vi "simon.vi"() -> ()   [LabVIEW 2021]
panel:
  out "Chaîne 4":string
  out "Gagné":bool
  out "Chaîne 3":string
  out "Chaîne 2":string
  in  "Cluster 3":T1
  in  "Pseudo":string
  out "Chaîne":string
  in  "Tableau":T2(array[cluster])
  in  "Tableau 3":T3(array[cluster])
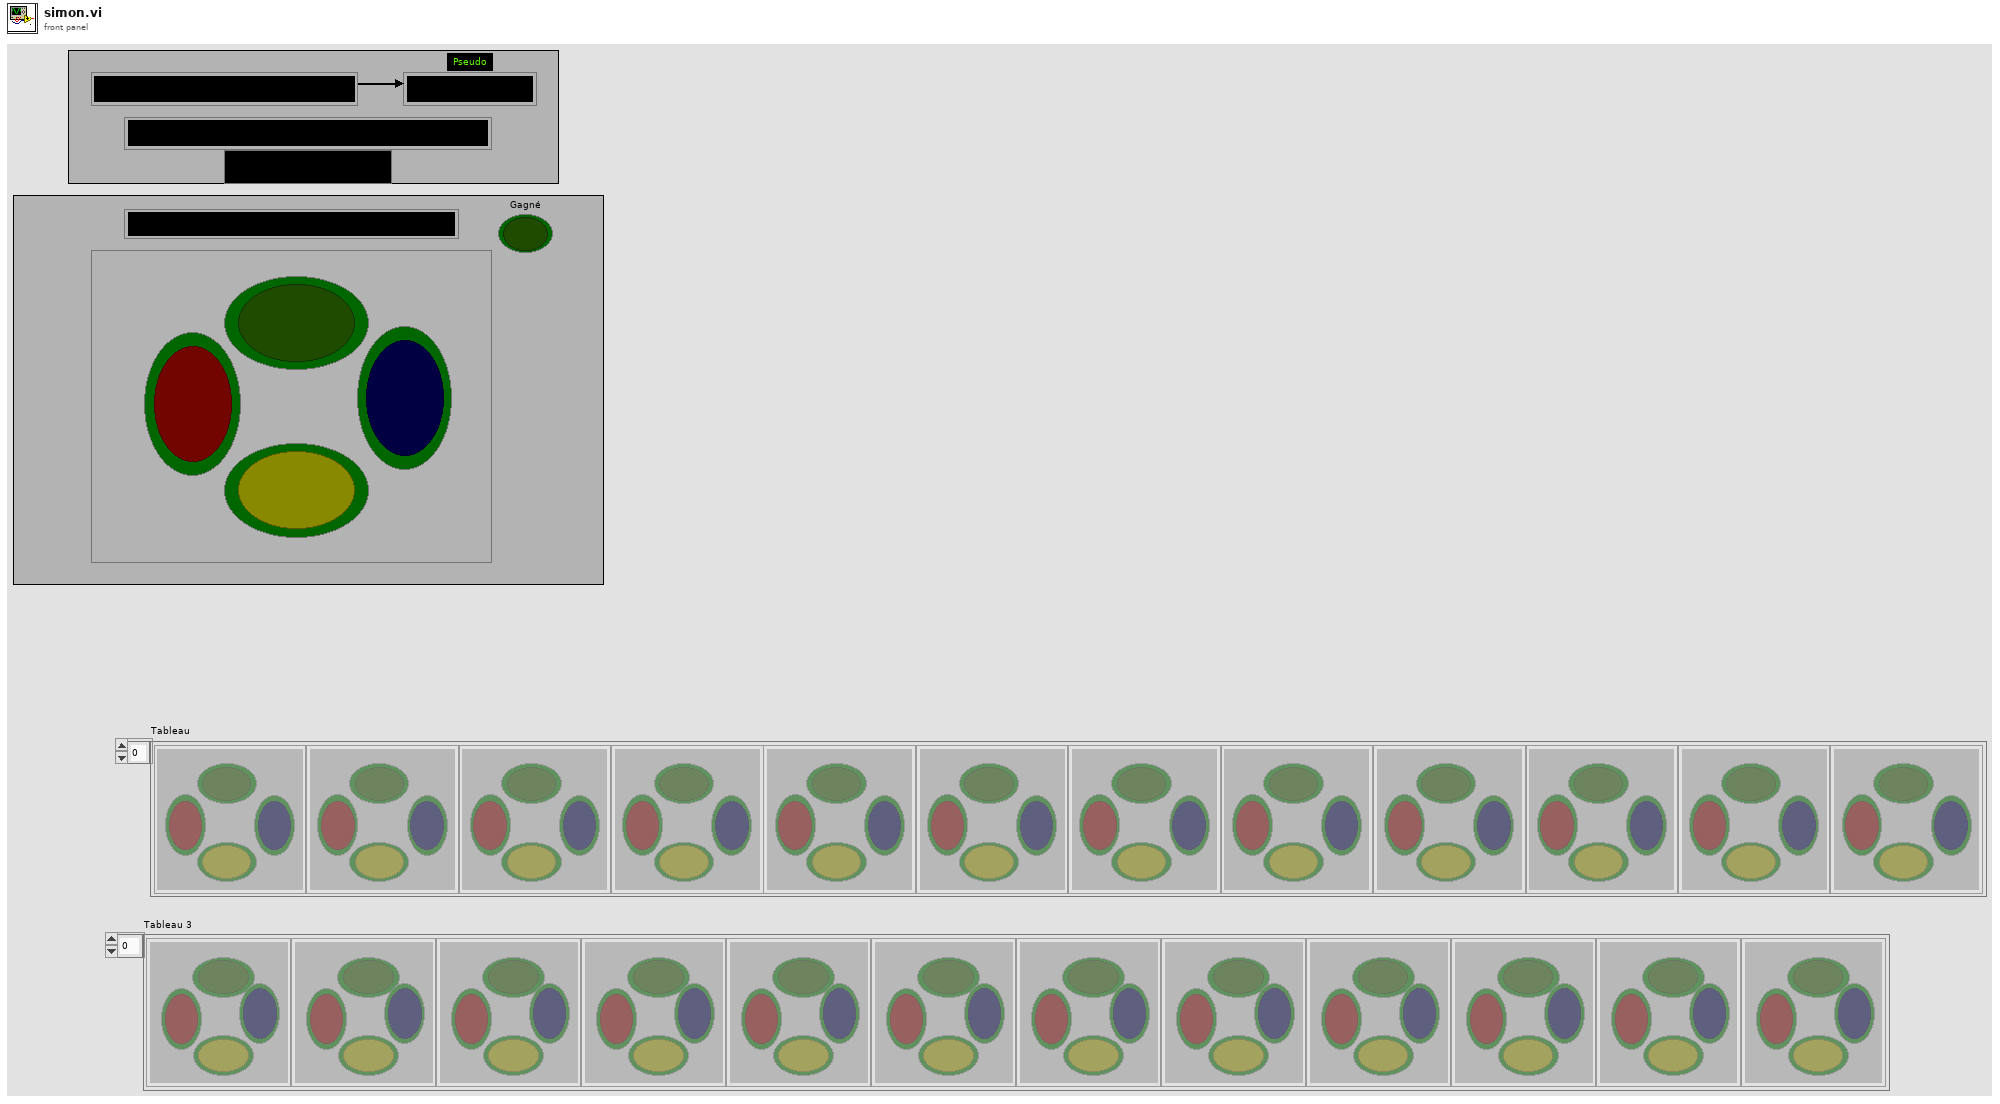
[diagram p1: front panel]
types:
  T1 = cluster{"Vert":bool, "Bleu":bool, "Rouge":bool, "Jaune":bool}
  T2 = cluster{"Vert":bool, "Bleu":bool, "Jaune":bool, "Rouge":bool}[]
  T3 = cluster{"Booléen":bool, "Booléen 2":bool, "Booléen 3":bool, "Booléen 4":bool}[]
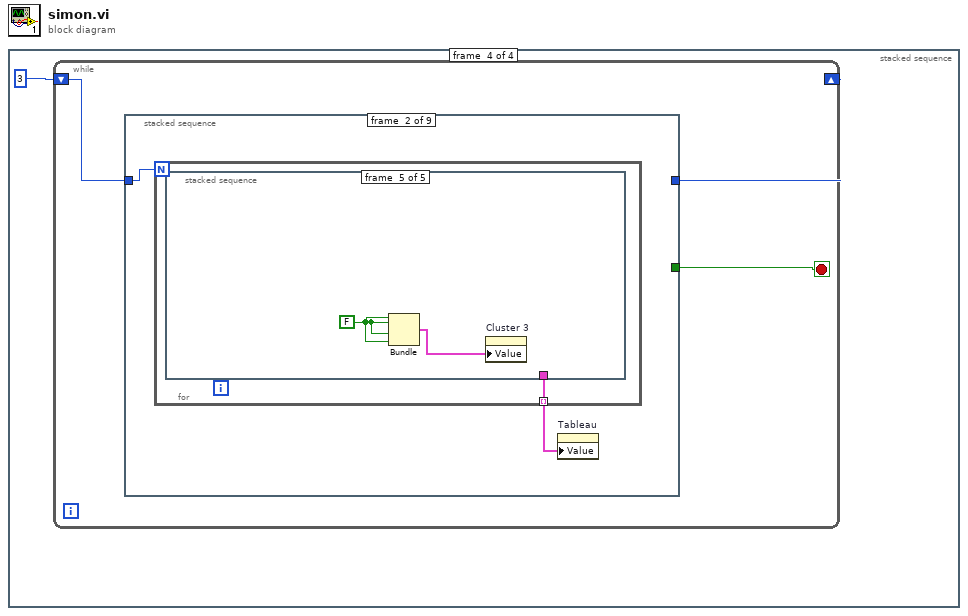
[diagram p0: block diagram]
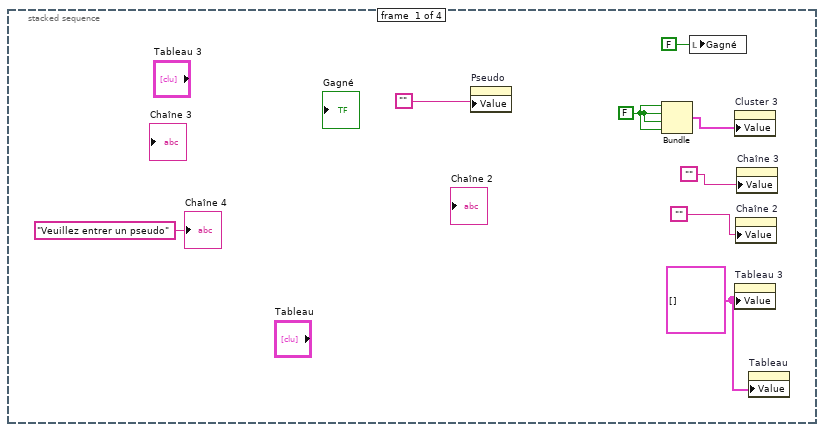
[diagram p2: hidden frame]
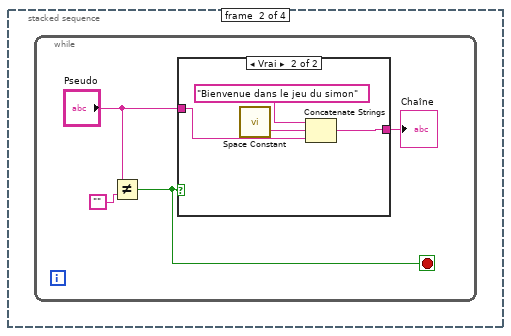
[diagram p3: hidden frame]
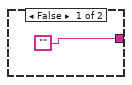
[diagram p4: hidden frame]
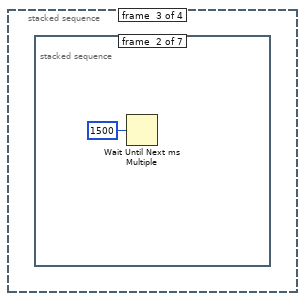
[diagram p5: hidden frame]
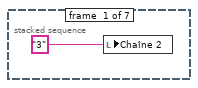
[diagram p6: hidden frame]
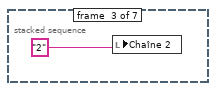
[diagram p7: hidden frame]
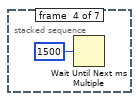
[diagram p8: hidden frame]
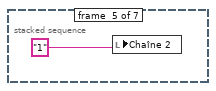
[diagram p9: hidden frame]
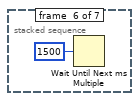
[diagram p10: hidden frame]
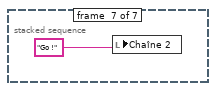
[diagram p11: hidden frame]
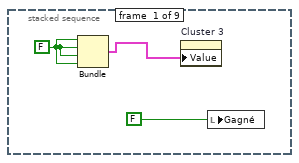
[diagram p12: hidden frame]
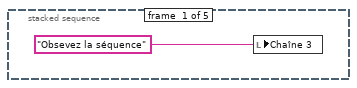
[diagram p13: hidden frame]
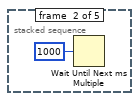
[diagram p14: hidden frame]
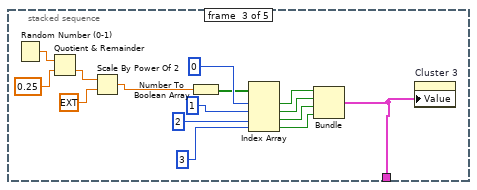
[diagram p15: hidden frame]
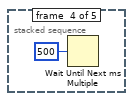
[diagram p16: hidden frame]
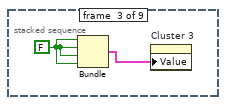
[diagram p17: hidden frame]
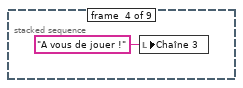
[diagram p18: hidden frame]
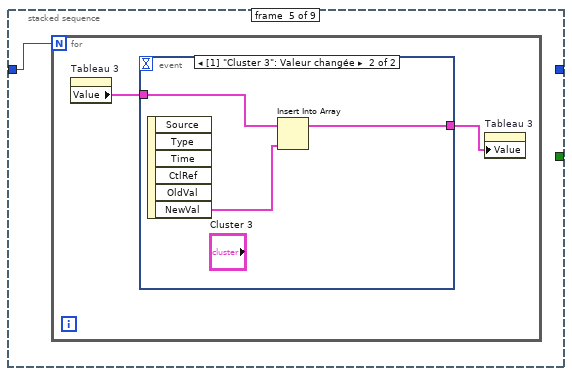
[diagram p19: hidden frame]
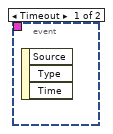
[diagram p20: hidden frame]
diagram:
  n1 = stacked-sequence {
    frame #0 {
      w3 = T3 [] ("Tableau 3")
      w7 = FALSE
      n2 = property on="Pseudo" class="Ch"("Value"="") -> ()  [unwired: 2 in, 2 out]
      n3 = Bundle(w7, w7, w7, w7) -> (w6:cluster{bool, bool, bool, bool})  [unwired: 1 in]
      n4 = local write "Gagné"(FALSE ("Booléen")) -> ()
      n5 = property on="Cluster 3" class="Clust"("Value"=w6) -> ()  [unwired: 2 in, 2 out]
      n6 = property on="Tableau 3" class="Tabl (strict)"("Value"=w3) -> ()  [unwired: 2 in, 2 out]
      n7 = property on="Chaîne 2" class="Ch"("Value"="") -> ()  [unwired: 2 in, 2 out]
      n8 = property on="Chaîne 3" class="Ch"("Value"="") -> ()  [unwired: 2 in, 2 out]
      n9 = property on="Tableau" class="Tabl (strict)"("Value"=w3) -> ()  [unwired: 2 in, 2 out]
      "Chaîne 4" <- "Veuillez entrer un pseudo" ("Chaîne 4")
    }
    frame #1 {
      n10 = while {
        stop <- w10 stop-if-true
        n11 = Not Equal?(x="Pseudo", y="") -> (x != y?=w10:bool)
        n12 = case shown="Vrai" w10 {
          tunnel: "Pseudo" -> [_ w14]
          tunnel: ["" w16] -> w12
          frame False {
          }
          frame True {
            n13 = call <vilib>:"Space Constant.vi"() -> ("String"=w15:string)
            n14 = Concatenate Strings("Bienvenue dans le jeu du simon", w15, w14) -> (w16:string)
          }
        }
        "Chaîne" <- w12
      }
    }
    frame #2 {
      n15 = stacked-sequence {
        frame #0 {
          n16 = local write "Chaîne 2"("3") -> ()
        }
        frame #1 {
          n17 = Wait Until Next ms Multiple(millisecond multiple=u32 1500 ("n millisecondes")) -> ()  [unwired: 1 out]
        }
        frame #2 {
          n18 = local write "Chaîne 2"("2") -> ()
        }
        frame #3 {
          n19 = Wait Until Next ms Multiple(millisecond multiple=u32 1500 ("n millisecondes")) -> ()  [unwired: 1 out]
        }
        frame #4 {
          n20 = local write "Chaîne 2"("1") -> ()
        }
        frame #5 {
          n21 = Wait Until Next ms Multiple(millisecond multiple=u32 1500 ("n millisecondes")) -> ()  [unwired: 1 out]
        }
        frame #6 {
          n22 = local write "Chaîne 2"("Go !") -> ()
        }
      }
    }
    frame #3 {
      n23 = while {
        shift-right: [w27] -> _
        shift-left: 3 -> [w28]
        stop <- w26 stop-if-true
        n24 = stacked-sequence {
          tunnel: w28 -> [_ w32 _ _ w58 w66 _ _ _]
          tunnel: [_ _ _ _ _ w65 _ _ _] -> w27
          tunnel: [_ _ _ _ _ _ w77 _ _] -> w26
          frame #0 {
            w31 = FALSE
            n25 = Bundle(w31, w31, w31, w31) -> (w30:cluster{bool, bool, bool, bool})  [unwired: 1 in]
            n26 = property on="Cluster 3" class="Clust"("Value"=w30) -> ()  [unwired: 2 in, 2 out]
            n27 = local write "Gagné"(FALSE) -> ()
          }
          frame #1 {
            n28 = for {
              N: w32 -> [_]
              tunnel: [w34] -> w33 mode=indexing
              n29 = stacked-sequence {
                tunnel: [_ _ w43 _ _] -> w34
                frame #0 {
                  n30 = local write "Chaîne 3"("Obsevez la séquence") -> ()
                }
                frame #1 {
                  n31 = Wait Until Next ms Multiple(millisecond multiple=u32 1000 ("n millisecondes")) -> ()  [unwired: 1 out]
                }
                frame #2 {
                  n32 = Random Number (0-1)() -> (number: 0 to 1=w41:dbl)
                  n33 = Quotient & Remainder(x=w41, y=0.25) -> (floor(x/y)=w39:dbl)  [unwired: 1 out]
                  n34 = Scale By Power Of 2(n=w39, x=ext 1.0) -> (x*2^n=w37:ext)
                  n35 = Number To Boolean Array(number=w37) -> (Boolean array=w38:bool[])
                  n36 = Index Array(array=w38, index #1=0 ("index"), index #2=1 ("index"), index #3=2 ("index"), index #4=3 ("index")) -> (element #1=w47:bool, element #2=w46:bool, element #3=w45:bool, element #4=w44:bool)
                  n37 = Bundle(w47, w46, w45, w44) -> (w43:cluster{bool, bool, bool, bool})  [unwired: 1 in]
                  n38 = property on="Cluster 3" class="Clust"("Value"=w43) -> ()  [unwired: 2 in, 2 out]
                }
                frame #3 {
                  n39 = Wait Until Next ms Multiple(millisecond multiple=u32 500 ("n millisecondes")) -> ()  [unwired: 1 out]
                }
                frame #4 {
                  w54 = FALSE
                  n40 = Bundle(w54, w54, w54, w54) -> (w53:cluster{bool, bool, bool, bool})  [unwired: 1 in]
                  n41 = property on="Cluster 3" class="Clust"("Value"=w53) -> ()  [unwired: 2 in, 2 out]
                }
              }
            }
            n42 = property on="Tableau" class="Tabl (strict)"("Value"=w33) -> ()  [unwired: 2 in, 2 out]
          }
          frame #2 {
            w56 = FALSE
            n43 = Bundle(w56, w56, w56, w56) -> (w55:cluster{bool, bool, bool, bool})  [unwired: 1 in]
            n44 = property on="Cluster 3" class="Clust"("Value"=w55) -> ()  [unwired: 2 in, 2 out]
          }
          frame #3 {
            n45 = local write "Chaîne 3"("A vous de jouer !" ("Chaîne 3")) -> ()
          }
          frame #4 {
            n46 = for {
              N: w58 -> [_]
              n47 = property on="Tableau 3" class="Tabl (strict)"() -> ("Value"=w60:T3)  [unwired: 2 in, 2 out]
              n48 = event shown="[1] \"Cluster 3\": Valeur changée" {
                selector: _ -> [_ _]
                dyn-events: _ -> [_ _]
                timeout: _ -> [_ _]
                tunnel: w60 -> [_ w63]
                tunnel: [_ w61] -> w59
                event Timeout {
                  n49 = event-data() -> ()  [unwired: 1 in, 3 out]
                }
                event "Cluster 3": Value Change {
                  n50 = event-data() -> ("NewVal"=w62:T1)  [unwired: 1 in, 5 out]
                  n51 = Insert Into Array(array=w63, new element=w62) -> (w61:T3)  [unwired: 1 in]
                }
              }
              n52 = property on="Tableau 3" class="Tabl (strict)"("Value"=w59) -> ()  [unwired: 2 in, 2 out]
            }
          }
          frame #5 {
            n53 = property on="Tableau 3" class="Tabl (strict)"() -> ("Value"=w69:T3)  [unwired: 2 in, 2 out]
            n54 = property on="Tableau" class="Tabl (strict)"() -> ("Value"=w68:T3)  [unwired: 2 in, 2 out]
            n55 = Equal?(x=w69, y=w68) -> (x = y?=w64:bool)
            n56 = case shown="Vrai" w64 {
              tunnel: [FALSE TRUE] -> w67
              tunnel: w66 -> [w70 w74]
              tunnel: [w70 w73] -> w65
              frame False {
                n57 = local write "Chaîne 3"("Perdu !" ("Chaîne 3")) -> ()
              }
              frame True {
                n58 = Increment(x=w74) -> (x+1=w73:i32)
                n59 = local write "Chaîne 3"("Gagné !") -> ()
              }
            }
            n60 = local write "Gagné"(w67) -> ()
          }
          frame #6 {
            n61 = property on="Gagné" class="Bool (strict)"() -> ("Value"=w78:bool)  [unwired: 2 in, 2 out]
            n62 = Equal?(x=w78, y=FALSE) -> (x = y?=w77:bool)
          }
          frame #7 {
            n63 = Wait Until Next ms Multiple(millisecond multiple=u32 1000 ("n millisecondes")) -> ()  [unwired: 1 out]
          }
          frame #8 {
            w81 = T3 [] ("Tableau 3")
            n64 = property on="Tableau" class="Tabl (strict)"("Value"=w81) -> ()  [unwired: 2 in, 2 out]
            n65 = property on="Tableau 3" class="Tabl (strict)"("Value"=w81) -> ()  [unwired: 2 in, 2 out]
          }
        }
      }
    }
  }
